vi "Do.vi"(8 "error in (no error)":errorcluster, 10 "Actor in":refnum<class "Actor.lvclass">, 11 "connect_to_controller Msg":refnum<class "connect_to_controller Msg.lvclass">) -> (0 "error out":errorcluster, 2 "Actor out":refnum<class "Actor.lvclass">)   [LabVIEW 2015, in "connect_to_controller Msg.lvclass"]
doc: "This VI delivers the message to the actor by calling the appropriate method(s) on the actor."
uses:
  connect_to_controller Msg.lvclass
  <vilib>/ActorFramework/Actor/Actor.lvclass
  xps_panel/newport_xps_panel.lvclass
  connect_to_controller Msg.lvclass/connect_to_controller Msg.ctl
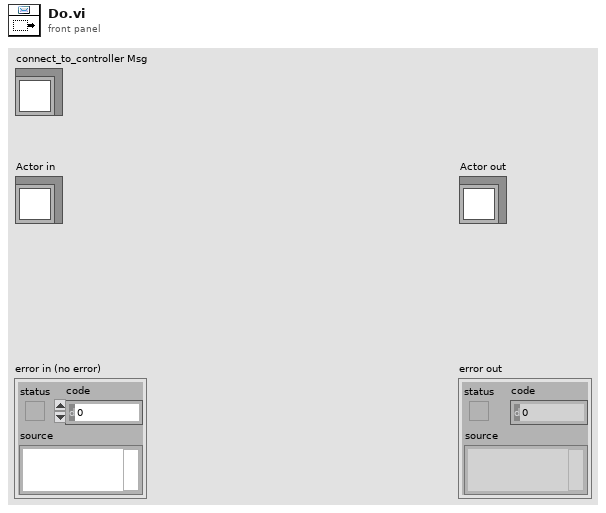
[diagram p1: front panel]
types:
  T1 = typedef "xps_login_info.ctl" = cluster{"IP Address":string, "User":string, "Password":string}
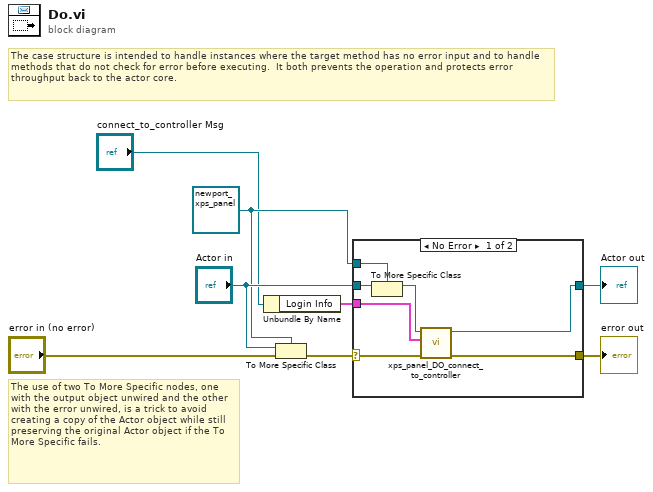
[diagram p0: block diagram]
diagram:
  w3 = refnum<class "newport_xps_panel.lvclass"> refnum ("Actor in")
  # "The use of two To More Specific nodes, one with the output object unwired and the other with the error unwired, is a trick to avoid creating a copy of the Actor object while still preserving the original Actor object if the To More Specific fails."
  # "The case structure is intended to handle instances where the target method has no error input and to handle methods that do not check for error before executing.  It both prevents the operation and protects error throughput back to the actor core."
  n1 = Unbundle By Name("connect_to_controller Msg") -> ("Login Info"=w1:T1)
  n2 = To More Specific Class(target class=w3, reference="Actor in", error in="error in (no error)") -> (error out=w7:errorcluster)  [unwired: 1 out]
  n3 = case shown="No Error" w7 {
    selector: w7 -> [w13 w17]
    tunnel: [w10 w17] -> w6
    tunnel: [w11 w16] -> w5
    tunnel: "Actor in" -> [w15 w16]
    tunnel: w3 -> [w14 _]
    tunnel: w1 -> [w9 _]
    frame No Error {
      n4 = To More Specific Class(target class=w14, reference=w15) -> (specific class reference=w12:refnum<class "newport_xps_panel.lvclass">)  [unwired: 1 in, 1 out]
      n5 = call "xps_panel_DO_connect_to_controller.vi"("error in (no error)"=w13, "Login Info"=w9, "newport_xps_panel in"=w12) -> ("error out"=w10:errorcluster, "newport_xps_panel out"=w11:refnum<class "newport_xps_panel.lvclass">)  [unwired: 7 in]
    }
    frame Error {
      # "If type check fails, pass the original object out again."
    }
  }
  "error out" <- w6
  "Actor out" <- w5
